vi "FinitCan.vi"(8 "错误输入（无错误）":errorcluster) -> (0 "错误输出":errorcluster)   [LabVIEW 2018]
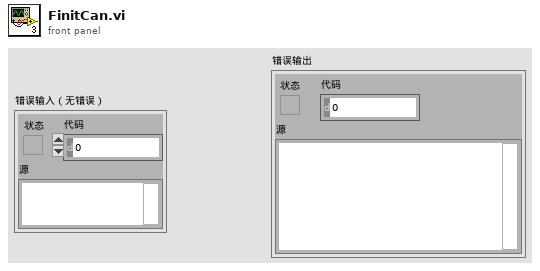
[diagram p1: front panel]
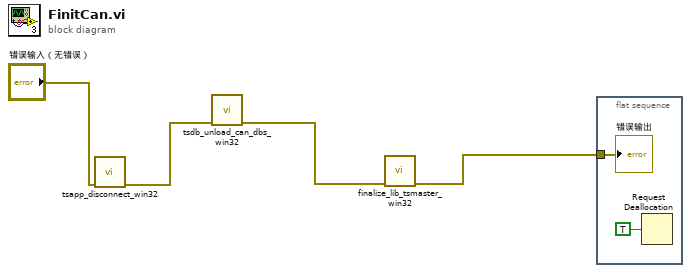
[diagram p0: block diagram]
diagram:
  n1 = call "tsapp_disconnect_win32.vi"("错误输入（无错误）"="错误输入（无错误）") -> ("错误输出"=w3:errorcluster)  [unwired: 8 in, 2 out]
  n2 = call "tsdb_unload_can_dbs_win32.vi"("错误输入（无错误）"=w3) -> ("错误输出"=w2:errorcluster)  [unwired: 9 in, 1 out]
  n3 = call "finalize_lib_tsmaster_win32.vi"("错误输入（无错误）"=w2) -> ("错误输出"=w4:errorcluster)  [unwired: 10 in]
  n4 = flat-sequence {
    tunnel: w4 -> [w6]
    frame #0 {
      n5 = Request Deallocation(TRUE ("标志")) -> ()
      "错误输出" <- w6
    }
  }
